vi "串口操作.vi"(0 "串口设置":T1={"COM号"="", "波特率"=9600, "数据比特"=8, "奇偶"=enum."None", "停止位"=10, "流控制"=0} {"流控制" items=["无"=0, "XON/XOFF"=1, "RTS/CTS"=2, "DTR/DSR"=4]; "停止位" items=["1.0"=10, "1.5"=15, "2.0"=20]; "数据比特" min=5 max=8 step=1; "波特率" items=["75"=75, "110"=110, "134"=134, "150"=150, "300"=300, "600"=600, "1200"=1200, "1800"=1800, "2400"=2400, "4800"=4800, "7200"=7200, "9600"=9600, "14400"=14400, "19200"=19200, "28800"=28800, "38400"=38400, "56000"=56000, "57600"=57600, "115200"=115200, "128000"=128000, "230400"=230400]}, 1 "错误输入（无错误）":errorcluster) -> (2 "输出最后的消息":string, 3 "当前串口号":refnum<visa-resource-name>, 4 "错误输出":errorcluster)   [LabVIEW 2015]
uses:
  Serial - Settings.ctl
panel:
  in  "消息缓冲":string
  out "消息提示":string
  in  "确定":bool
  in  "打开":bool
  out "预设串口号":refnum<visa-resource-name>
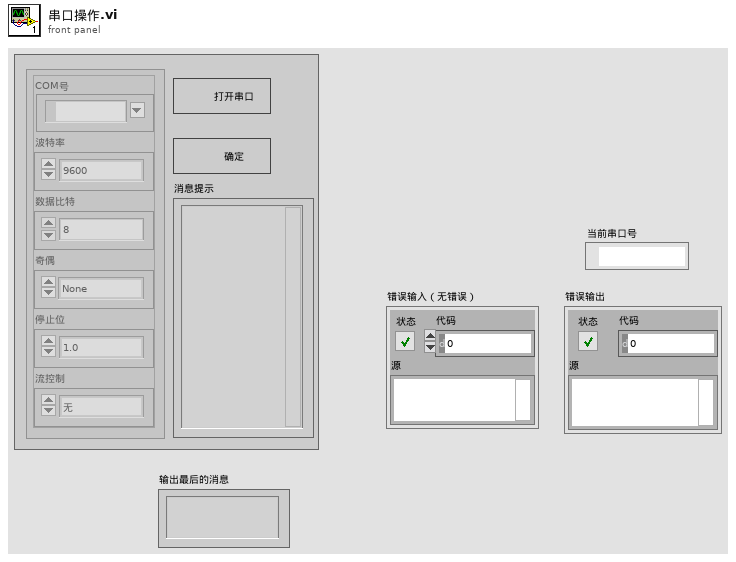
[diagram p1: front panel]
types:
  T1 = typedef "Serial - Settings.ctl" = cluster{"COM号":refnum<visa-resource-name>, "波特率":u32, "数据比特":u16, "奇偶":enum16{"None", "Odd", "Even", "Mark", "Space"}, "停止位":u16, "流控制":u16}
  T2 = typedef "串口操作函数状态机枚举.ctl" = enum16{"初始化", "等待按键", "串口打开", "串口关闭", "提示消息", "退出"}
  T3 = enum8{"Enabled", "Disabled", "Disabled and Grayed Out"}
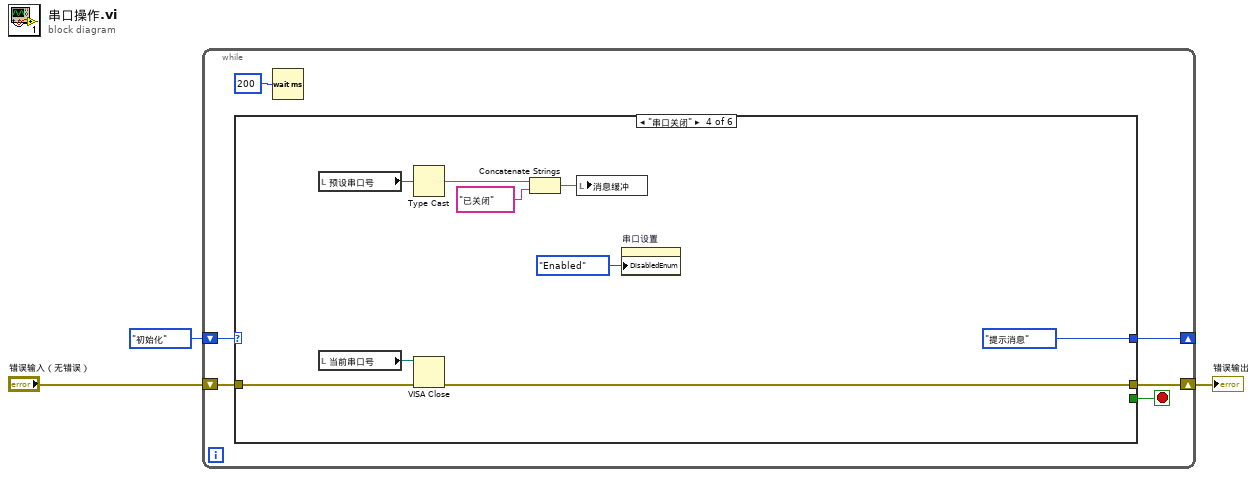
[diagram p0: block diagram]
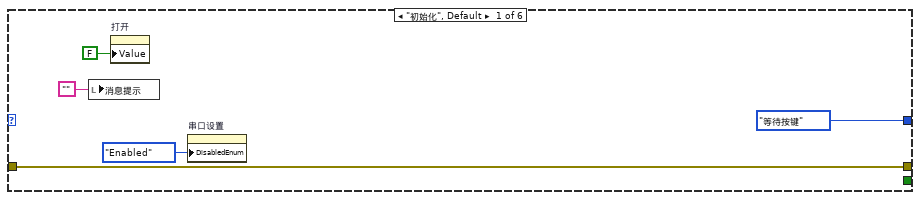
[diagram p2: hidden frame]
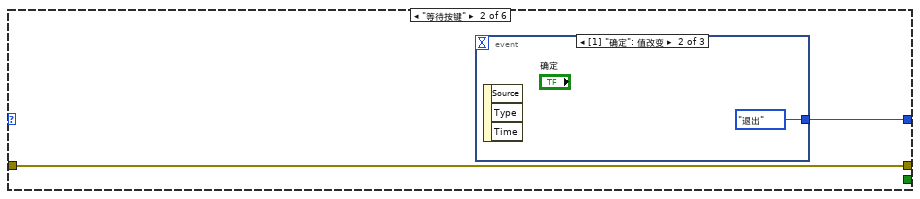
[diagram p3: hidden frame]
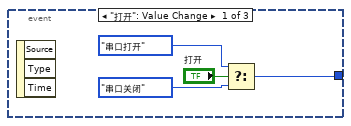
[diagram p4: hidden frame]
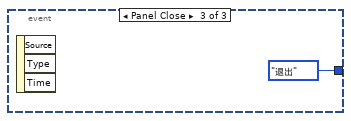
[diagram p5: hidden frame]
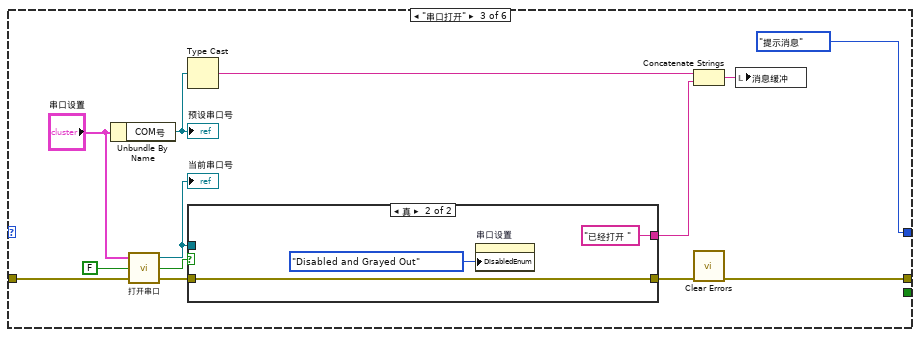
[diagram p6: hidden frame]
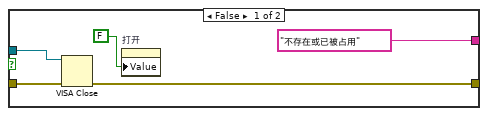
[diagram p7: hidden frame]
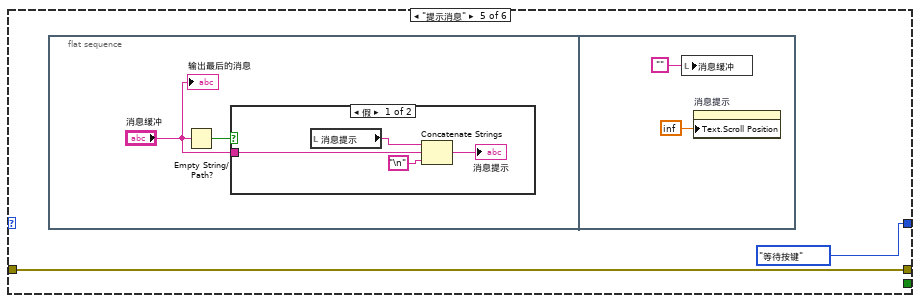
[diagram p8: hidden frame]
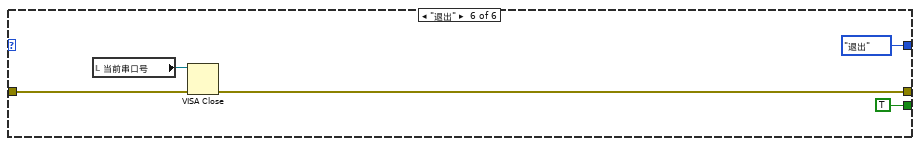
[diagram p10: hidden frame]
diagram:
  n1 = while {
    shift-right: [w4] -> w2
    shift-left: "错误输入（无错误）" -> [w5]
    shift-right: [w6] -> _
    shift-left: 串口操作函数状态机枚举."初始化" -> [w8]
    stop <- w7 stop-if-true
    n2 = case shown="\"串口关闭\"" w8 {
      tunnel: [_ _ _ _ _ TRUE ("退出")] -> w7
      tunnel: [串口操作函数状态机枚举."等待按键" w16 串口操作函数状态机枚举."提示消息" 串口操作函数状态机枚举."提示消息" 串口操作函数状态机枚举."等待按键" 串口操作函数状态机枚举."退出"] -> w6
      tunnel: w5 -> [w12 w15 w27 w47 w53 w64]
      tunnel: [w12 w15 w31 w46 w53 w63] -> w4
      frame "初始化", Default {
        n3 = local write "消息提示"("") -> ()
        n4 = property on="打开" class="Bool (严格)"("Value"=FALSE ("打开")) -> ()  [unwired: 2 in, 2 out]
        n5 = property on="串口设置" class="Clust (严格)"("DisabledEnum"=T3."Enabled" ("禁用")) -> ()  [unwired: 2 in, 2 out]
      }
      frame "等待按键" {
        n6 = event shown="[1] \"确定\": 值改变" {
          selector: _ -> [_ _ _]
          dyn-events: _ -> [_ _ _]
          timeout: _ -> [_ _ _]
          tunnel: [w18 串口操作函数状态机枚举."退出" 串口操作函数状态机枚举."退出"] -> w16
          event "打开": Value Change {
            n7 = event-data() -> ()  [unwired: 1 in, 3 out]
            n8 = Select(t=串口操作函数状态机枚举."串口打开", s="打开", f=串口操作函数状态机枚举."串口关闭") -> (s? t:f=w18:T2)
          }
          event "确定": Value Change {
            n9 = event-data() -> ()  [unwired: 1 in, 3 out]
          }
          event Panel Close {
            n10 = event-data() -> ()  [unwired: 1 in, 3 out]
          }
        }
      }
      frame "串口打开" {
        n11 = Unbundle By Name("串口设置") -> ("COM号"=w34:refnum<visa-resource-name>)
        "预设串口号" <- w34
        n12 = call "打开串口.vi"("错误输入（无错误）"=w27, "是否对话框提示？"=FALSE, "串口设置"="串口设置") -> ("错误输出"=w26:errorcluster, "OpenOK?"=w25:bool, "VISA引用句柄输出"=w24:refnum<visa-resource-name>)
        "当前串口号" <- w24
        n13 = Type Cast(x=w34) -> (*(type *) &x=w33:string)  [unwired: 1 in]
        n14 = case shown="真" w25 {
          tunnel: ["不存在或已被占用" "已经打开 "] -> w32
          tunnel: w24 -> [w39 _]
          tunnel: w26 -> [w38 w42]
          tunnel: [w37 w42] -> w35
          frame False {
            n15 = VISA Close(VISA resource name=w39, error in (no error)=w38) -> (error out=w37:errorcluster)
            n16 = property on="打开" class="Bool (严格)"("Value"=FALSE ("打开")) -> ()  [unwired: 2 in, 2 out]
          }
          frame True {
            n17 = property on="串口设置" class="Clust (严格)"("DisabledEnum"=T3."Disabled and Grayed Out" ("禁用")) -> ()  [unwired: 2 in, 2 out]
          }
        }
        n18 = Concatenate Strings(w33, w32) -> (w29:string)
        n19 = call <vilib>:"Clear Errors.vi"("error in (no error)"=w35) -> ("error out"=w31:errorcluster)  [unwired: 5 in, 1 out]
        n20 = local write "消息缓冲"(w29) -> ()
      }
      frame "串口关闭" {
        n21 = local read "预设串口号"() -> (w51:refnum<visa-resource-name>)
        n22 = local read "当前串口号"() -> (w52:refnum<visa-resource-name>)
        n23 = Type Cast(x=w51) -> (*(type *) &x=w49:string)  [unwired: 1 in]
        n24 = VISA Close(VISA resource name=w52, error in (no error)=w47) -> (error out=w46:errorcluster)
        n25 = Concatenate Strings(w49, "已关闭") -> (w45:string)
        n26 = local write "消息缓冲"(w45) -> ()
        n27 = property on="串口设置" class="Clust (严格)"("DisabledEnum"=T3."Enabled" ("禁用")) -> ()  [unwired: 2 in, 2 out]
      }
      frame "提示消息" {
        n28 = flat-sequence {
          frame #0 {
            n29 = Empty String/Path?(string/path="消息缓冲") -> (empty?=w56:bool)
            n30 = case shown="假" w56 {
              tunnel: "消息缓冲" -> [w59 _]
              frame False {
                n31 = local read "消息提示"() -> (w58:string)
                n32 = Concatenate Strings(w58, w59, "\n") -> (→"消息提示":string)
              }
              frame True {
              }
            }
            "输出最后的消息" <- "消息缓冲"
          }
          frame #1 {
            n33 = local write "消息缓冲"("") -> ()
            n34 = property on="消息提示" class="Str"("Text.Scroll Position"=inf) -> ()  [unwired: 2 in, 2 out]
          }
        }
      }
      frame "退出" {
        n35 = local read "当前串口号"() -> (w65:refnum<visa-resource-name>)
        n36 = VISA Close(VISA resource name=w65, error in (no error)=w64) -> (error out=w63:errorcluster)
      }
    }
    n37 = Wait (ms)(milliseconds to wait=u32 200 ("等待时间（毫秒）")) -> ()  [unwired: 1 out]
  }
  "错误输出" <- w2
